vi "Multipart reply - simple.vi"() -> ()   [LabVIEW 2015]
uses:
  <vilib>/addons/zeromq/socket_type.ctl
  <vilib>/addons/zeromq/zmq_context.lvclass
  <vilib>/addons/zeromq/zmq_socket.lvclass
  <vilib>/addons/zeromq/zeromq.lvlib
panel:
  in  "stop":bool
  out "error out":errorcluster
  in  "endpoint":string="tcp://127.0.0.1:5555"
  out "data received":string[](array[string])
  # "ZeroMQ Multipart reply VI - simple"
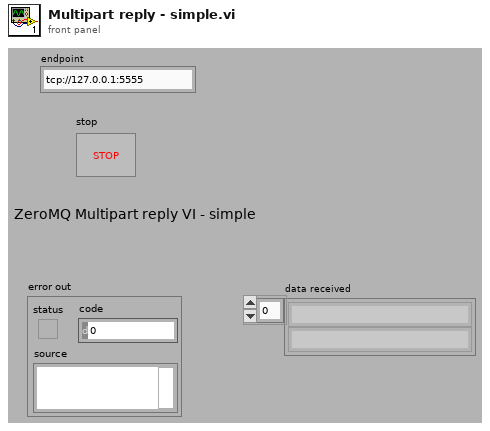
[diagram p1: front panel]
types:
  T1 = typedef "zeromq.lvlib/socket_type.ctl" = enum8{"ZMQ_PAIR", "ZMQ_PUB", "ZMQ_SUB", "ZMQ_REQ", "ZMQ_REP", "ZMQ_DEALER", "ZMQ_ROUTER", "ZMQ_PULL", "ZMQ_PUSH", "ZMQ_XPUB", "ZMQ_XSUB"}
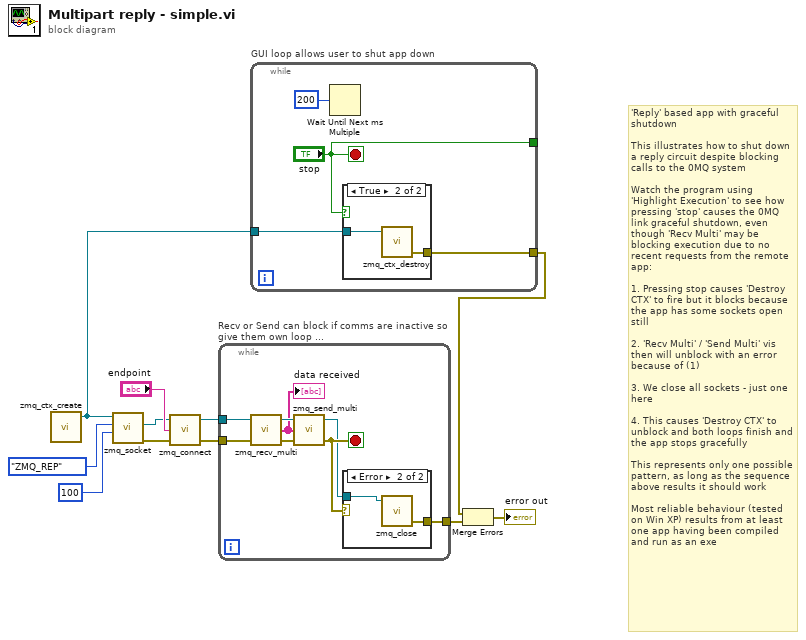
[diagram p0: block diagram]
diagram:
  # "'Reply' based app with graceful shutdown\n\nThis illustrates how to shut down a reply circuit despite blocking calls to the 0MQ system\n\nWatch the program using 'Highlight Execution' to see how pressing 'stop' causes the 0MQ link graceful shutdown, even though 'Recv Multi' may be blocking execution due to no recent requests from the remote app:\n\n1. Pressing stop causes 'Destroy CTX' to fire but it blocks because the app has some sockets open still\n\n2. 'Recv Multi' / 'Send Multi' vis then will unblock with an error because of (1)\n\n3. We close all sockets - just one here\n\n4. This causes 'Destroy CTX' to unblock and both loops finish and the app stops gracefully\n\nThis represents only one possible pattern, as long as the sequence above results it should work\n\nMost reliable behaviour (tested on Win XP) results from at least one app having been compiled and run as an exe"
  n1 = call <vilib>:"zmq_ctx_create.vi"() -> ("context out"=w1:refnum<class "zmq_context.lvclass">)  [unwired: 4 in, 1 out]
  n2 = call <vilib>:"zmq_socket.vi"("linger (ms)"=100, "socket type"=socket_type."ZMQ_REP", "context in"=w1) -> ("error out"=w6:errorcluster, "socket out"=w2:refnum<class "zmq_socket.lvclass">)  [unwired: 2 in, 1 out]
  n3 = call <vilib>:"zmq_connect.vi"("error in"=w6, "endpoint"="endpoint", "socket in"=w2) -> ("error out"=w5:errorcluster, "socket out"=w4:refnum<class "zmq_socket.lvclass">)  [unwired: 1 in]
  n4 = while "Recv or Send can block if comms are inactive so give them own loop ..." {
    tunnel: [w14] -> w7
    tunnel: w5 -> [w13]
    tunnel: w4 -> [w12]
    stop <- w16 stop-if-true
    n5 = call <vilib>:"zmq_recv_multi.vi"("error in"=w13, "socket in"=w12) -> ("error out"=w18:errorcluster, "parts"=w17:string[], "socket out"=w19:refnum<class "zmq_socket.lvclass">)  [unwired: 1 in]
    "data received" <- w17
    n6 = call <vilib>:"zmq_send_multi.vi"("error in"=w18, "parts"=w17, "socket in"=w19) -> ("error out"=w16:errorcluster, "socket out"=w15:refnum<class "zmq_socket.lvclass">)  [unwired: 1 in]
    n7 = case shown="Error" w16 {
      tunnel: w15 -> [_ w21]
      tunnel: [_ w20] -> w14
      frame No Error {
      }
      frame Error {
        n8 = call <vilib>:"zmq_close.vi"("socket"=w21) -> ("error out"=w20:errorcluster)  [unwired: 4 in]
      }
    }
  }
  n9 = while "GUI loop allows user to shut app down" {
    tunnel: w1 -> [w25]
    tunnel: [w24] -> w8
    tunnel: ["stop"] -> _
    stop <- "stop" stop-if-true
    n10 = Wait Until Next ms Multiple(millisecond multiple=u32 200) -> ()  [unwired: 1 out]
    n11 = case shown="True" "stop" {
      tunnel: w25 -> [_ w26]
      tunnel: [_ w27] -> w24
      frame False {
      }
      frame True {
        n12 = call <vilib>:"zmq_ctx_destroy.vi"("context in"=w26) -> ("error out"=w27:errorcluster)  [unwired: 4 in]
      }
    }
  }
  n13 = Merge Errors(w8, w7) -> (→"error out":errorcluster)
